vi "AddClasses.vi"(0 "reference in":refnum<class "Executer.lvclass">, 2 "Classes":refnum<class>[](array[class]), 5 "error in (no error)":errorcluster) -> (14 "reference out":refnum<class "Executer.lvclass">, 19 "error out":errorcluster)   [LabVIEW 2018, in "Executer.lvclass"]
uses:
  Executer.lvclass
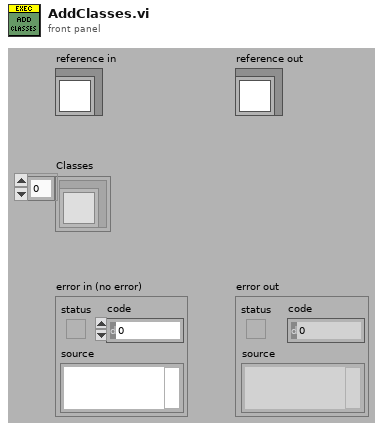
[diagram p1: front panel]
types:
  T1 = typedef "Executer.lvclass/ClassExecutionInfo.ctl" = cluster{"Class":refnum<class>, "ClassName":string, "VIExecutionInfo":T2[]}
  T2 = typedef "Executer.lvclass/MethodExecutionInfo.ctl" = cluster{"viRef":refnum<vi>, "MethodName":string, "ControlIndices":i32[], "ClassInIndex":i32, "IndicatorIndices":i32[], "ErrorOutIndex":i32, "ControlTypes":variant[]}
  T3 = typedef "Executer.lvclass/ObjectAttributes.ctl" = cluster{"Executions":T1[]}
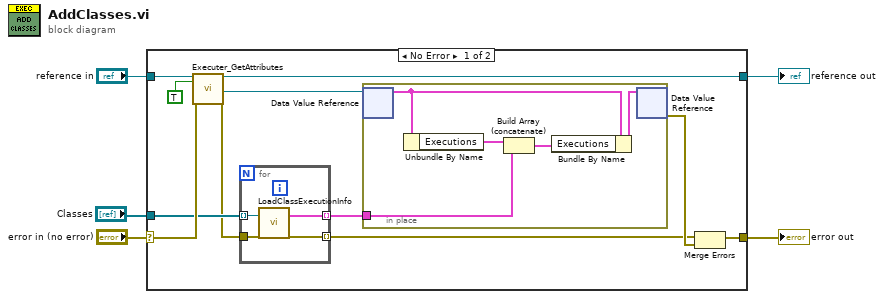
[diagram p0: block diagram]
diagram:
  n1 = case shown="No Error" "error in (no error)" {
    selector: "error in (no error)" -> [w13 w27]
    tunnel: [w15 w27] -> w4
    tunnel: [w11 w26] -> w2
    tunnel: "reference in" -> [w14 w26]
    tunnel: "Classes" -> [w9 _]
    frame No Error {
      n2 = call "Executer_GetAttributes.vi"("reference in"=w14, "OnlyGetDvrReference(False)"=TRUE, "error in (no error)"=w13) -> ("reference out"=w11:refnum<class "Executer.lvclass">, "DataRef"=w12:refnum<data-value>, "error out"=w8:errorcluster)  [unwired: 13 in, 1 out]
      n3 = for {
        tunnel: w9 -> [w20] mode=indexing
        tunnel: [w18] -> w7 mode=indexing
        tunnel: w8 -> [w19]
        tunnel: [w17] -> w6 mode=indexing
        n4 = call "LoadClassExecutionInfo.vi"("class in"=w20, "error in (no error)"=w19) -> ("ClassExecutionInfo"=w18:T1, "error out"=w17:errorcluster)  [unwired: 16 in]
      }
      n5 = in-place {
        in-place-border: w7 -> [w21]
        n6 = in-place-dvr #1(w12) -> (w24:T3)  [unwired: 1 out]
        n7 = Unbundle By Name(w24) -> ("Executions"=w23:T1[])
        n8 = Build Array (concatenate)(w23, w21) -> (w22:T1[])
        n9 = Bundle By Name(cluster=w24, "Executions"=w22) -> (w25:T3)
        n10 = in-place-dvr #1(w25) -> (w16:errorcluster)  [unwired: 1 out]
      }
      n11 = Merge Errors(w6, w16) -> (w15:errorcluster)
    }
    frame Error {
    }
  }
  "error out" <- w4
  "reference out" <- w2
